vi "Zero Displacement.vi"(7 "Device Number":T1, 10 "Zero":bool) -> ()   [LabVIEW 2016]
uses:
  _TypeDefs/FRIC_navX_DeviceNumbersTypeDef.ctl
  _TypeDefs/Z900_navX_ActionTypeDef.ctl
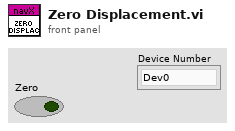
[diagram p1: front panel]
types:
  T1 = typedef "FRIC_navX_DeviceNumbersTypeDef.ctl" = enum16{"Dev0", "Dev1", "Dev2", "Dev3"}
  T2 = typedef "Z900_navX_ActionTypeDef.ctl" = enum16{"None", "Halt", "Normal Read", "Update Serial Protocol", "Update Rate Htz", "Zero-Yaw", "Zero-Displacement", "Zero-Velocity"}
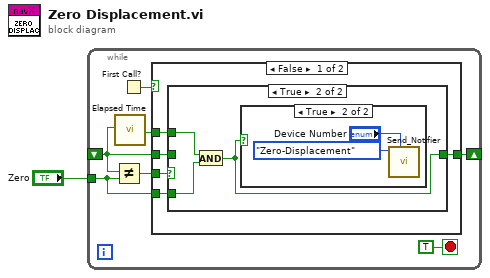
[diagram p0: block diagram]
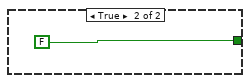
[diagram p4: hidden frame]
diagram:
  n1 = while {
    shift-right: [w7] -> _
    shift-left: _ -> [w3]
    tunnel: "Zero" -> [w4]
    stop <- TRUE stop-if-true
    n2 = Not Equal?(x=w3, y=w4) -> (x != y?=w6:bool)
    n3 = call "Elapsed Time"("Reset"=w3) -> ("Time has Elapsed"=w2:bool)  [unwired: 11 in, 7 out]
    n4 = First Call?() -> (First Call?: T/F=w5:bool)
    n5 = case shown="False" w5 {
      tunnel: [w13 FALSE] -> w7
      tunnel: w3 -> [w12 _]
      tunnel: w6 -> [w11 _]
      tunnel: w4 -> [w10 _]
      tunnel: w2 -> [w9 _]
      frame False {
        n6 = case shown="True" w11 {
          tunnel: [w14 w15] -> w13
          tunnel: w12 -> [w14 _]
          tunnel: w10 -> [_ w16]
          tunnel: w9 -> [_ w17]
          frame False {
          }
          frame True {
            n7 = And(x=w17, y=w16) -> (x .and. y?=w15:bool)
            n8 = case shown="True" w15 {
              frame False {
              }
              frame True {
                n9 = call "Send_Notifier.vi"("Device Number"="Device Number", "navX Action"=Z900_navX_ActionTypeDef."Zero-Displacement") -> ()  [unwired: 10 in]
              }
            }
          }
        }
      }
      frame True {
      }
    }
  }
